vi "Wago Room PID Settings.vi"(8 "Error In":errorcluster, 10 "Wago Data Input":T2 {"Input Process Image"."Software Constants"."Room PID Settings"."Room Dehumid Temperature I (*RM Dehum I1)" max=30000 step=1; "Input Process Image"."Software Constants"."Room PID Settings"."Room Dehumid Temperature P (*RM Dehum P1)" max=30000 step=1; "Input Process Image"."Software Constants"."Room PID Settings"."Room Cool Temperature I (*RM Cool I1)" max=30000 step=1; "Input Process Image"."Software Constants"."Room PID Settings"."Room Cool Temperature P (*RM Cool P1)" max=30000 step=1; "Input Process Image"."Software Constants"."Room PID Settings"."Room Heat I (*RM Heat I1)" max=30000 step=1; "Input Process Image"."Software Constants"."Room PID Settings"."Room Heat P (*RM Heat P1)" max=30000 step=1; "Input Process Image"."Software Constants"."Room PID Settings"."Room Humidity I (*RM Hum I1)" max=30000 step=1; "Input Process Image"."Software Constants"."Room PID Settings"."Room Humidity P (*RM Hum P1)" max=30000 step=1; "Input Process Image"."Software Constants"."Room PID Settings"."Room Dry I (*RM Dry I1)" max=30000 step=1; "Input Process Image"."Software Constants"."Room PID Settings"."Room Dry P(*RM Dry P1)" max=30000 step=1}, 11 "Modbus Master in":refnum<class "Modbus Master.lvclass">) -> (0 "Error Out":errorcluster, 2 "Wago Data Output":T2 {"Input Process Image"."Software Constants"."Room PID Settings"."Room Dehumid Temperature I (*RM Dehum I1)" max=30000 step=1; "Input Process Image"."Software Constants"."Room PID Settings"."Room Dehumid Temperature P (*RM Dehum P1)" max=30000 step=1; "Input Process Image"."Software Constants"."Room PID Settings"."Room Cool Temperature I (*RM Cool I1)" max=30000 step=1; "Input Process Image"."Software Constants"."Room PID Settings"."Room Cool Temperature P (*RM Cool P1)" max=30000 step=1; "Input Process Image"."Software Constants"."Room PID Settings"."Room Heat I (*RM Heat I1)" max=30000 step=1; "Input Process Image"."Software Constants"."Room PID Settings"."Room Heat P (*RM Heat P1)" max=30000 step=1; "Input Process Image"."Software Constants"."Room PID Settings"."Room Humidity I (*RM Hum I1)" max=30000 step=1; "Input Process Image"."Software Constants"."Room PID Settings"."Room Humidity P (*RM Hum P1)" max=30000 step=1; "Input Process Image"."Software Constants"."Room PID Settings"."Room Dry I (*RM Dry I1)" max=30000 step=1; "Input Process Image"."Software Constants"."Room PID Settings"."Room Dry P(*RM Dry P1)" max=30000 step=1}, 3 "Modbus Master out":refnum<class "Modbus Master.lvclass">)   [LabVIEW 2016]
uses:
  <vilib>/NI/Modbus Library/API/Master/Modbus Master.lvclass
  Type Definitions/Wago Main Control.ctl
  Type Definitions/Wago Output Data Process Image.ctl
  Type Definitions/Wago Room Condtions.ctl
  Type Definitions/Wago Door Relays.ctl
  Type Definitions/Wago Contactor Settings.ctl
  Type Definitions/Wago Ground Leakage.ctl
  Type Definitions/Wago Input Process Image.ctl
  Type Definitions/Wago Room PID Settings.ctl
  Type Definitions/Wago Measured Input Data.ctl
  Type Definitions/Wago Room Setpoint Targets.ctl
  Type Definitions/Wago Input Commands.ctl
panel:
  in  "Ring 10":T1=344 items=["fwS1Volt1"=0, "fwS1Volt2"=1, "fwS2Volt1"=2, "fwS2Volt2"=3, "fwS3Volt1"=4, "fwS3Volt2"=5, "fwS4Volt1"=6, "fwS4Volt2"=7, "fwS5Volt1"=8, "fwS5Volt2"=9, "fwS6Volt1"=10, "fwS6Volt2 "=11, "fwS7Volt1"=12, "fwS7Volt2"=13, "fwS8Volt1"=14, "fwS8Volt2"=15, "fwRoomHum"=16, "fwRoomTemp"=17, "fwAISpare1"=18, "fwAISpare2"=19, "fwSuppTemp"=20, "fwCoolTemp"=21, "fwDehumTemp"=22, "fwUnused"=23, "Bool Inputs"=24, "gwVoltRate1"=256, "gwVoltRate2"=257, "gwVoltRate3"=258, "gwVoltRate4"=259, "gwVoltRate5"=260, "gwVoltRate6"=261, "gwVoltRate7"=262, "gwVoltRate8"=263, "gwVoltWindow5/1"=264, "gwVoltWindow6/2"=265, "gwVoltWindow7/3"=266, "gwVoltWindow8/4"=267, "fwVoltSet1"=272, "fwVoltSet2"=273, "fwVoltSet3"=274, "fwVoltSet4"=275, "fwVoltSet5"=276, "fwVoltSet6"=277, "fwVoltSet7"=278, "fwVoltSet8"=279, "fwVoltRng1"=280, "fwVoltRng2"=281, "fwVoltRng3"=282, "fwVoltRng4"=283, "fwVoltRng5"=284, "fwVoltRng6"=285, "fwVoltRng7"=286, "fwVoltRng8"=287, "fwVoltPol1"=296, "fwVoltPol2"=297, "fwVoltPol3"=298, "fwVoltPol4"=299, "fwVoltPol5"=300, "fwVoltPol6"=301, "fwVoltPol7"=302, "fwVoltPol8"=303, "Rm1St1Dr1Cmd"=304, "Rm1St2Dr1Cmd"=305, "Rm1St3Dr1Cmd"=306, "Rm1St4Dr1Cmd"=307, "Rm1St5Dr1Cmd"=308, "Rm1St6Dr1Cmd"=309, "Rm1St7Dr1Cmd"=310, "Rm1St8Dr1Cmd"=311, "Rm1St1Dr2Cmd"=312, "Rm1St2Dr2Cmd"=313, "Rm1St3Dr2Cmd"=314, "Rm1St4Dr2Cmd"=315, "Rm1St5Dr2Cmd"=316, "Rm1St6Dr2Cmd"=317, "Rm1St7Dr2Cmd"=318, "Rm1St8Dr2Cmd"=319, "Rm1St1Dr3Cmd"=320, "Rm1St2Dr3Cmd"=321, "Rm1St3Dr3Cmd"=322, "Rm1St4Dr3Cmd"=323, "Rm1St5Dr3Cmd"=324, "Rm1St6Dr3Cmd"=325, "Rm1St7Dr3Cmd"=326, "Rm1St8Dr3Cmd"=327, "fwRmTempSP"=328, "fwRmHumSP"=329, "fwCoolTempSP"=330, "fwDehumTempSP"=331, "fwRmRun"=332, "fwRmOk"=333, "fwTesting"=334, "fwRmDryP"=335, "fwRmDryI"=336, "fwRmHumP"=337, "fwRmHumI"=338, "fwRmHeatP"=339, "fwRmHeatI"=340, "fwCoolTempP"=341, "fwCoolTempI"=342, "fwDehumTempP"=343, "fwDehumTempI"=344, "fwGndLeak1"=345, "fwGndLeak2"=346, "fwGndLeak3"=347, "fwGndLeak4"=348, "fwGndLeak5"=349, "fwGndLeak6"=350, "fwGndLeak7"=351, "fwGndLeak8"=352, "Rm1OpenerCmd"=353]
  in  "Ring 9":T1=343 items=["fwS1Volt1"=0, "fwS1Volt2"=1, "fwS2Volt1"=2, "fwS2Volt2"=3, "fwS3Volt1"=4, "fwS3Volt2"=5, "fwS4Volt1"=6, "fwS4Volt2"=7, "fwS5Volt1"=8, "fwS5Volt2"=9, "fwS6Volt1"=10, "fwS6Volt2 "=11, "fwS7Volt1"=12, "fwS7Volt2"=13, "fwS8Volt1"=14, "fwS8Volt2"=15, "fwRoomHum"=16, "fwRoomTemp"=17, "fwAISpare1"=18, "fwAISpare2"=19, "fwSuppTemp"=20, "fwCoolTemp"=21, "fwDehumTemp"=22, "fwUnused"=23, "Bool Inputs"=24, "gwVoltRate1"=256, "gwVoltRate2"=257, "gwVoltRate3"=258, "gwVoltRate4"=259, "gwVoltRate5"=260, "gwVoltRate6"=261, "gwVoltRate7"=262, "gwVoltRate8"=263, "gwVoltWindow5/1"=264, "gwVoltWindow6/2"=265, "gwVoltWindow7/3"=266, "gwVoltWindow8/4"=267, "fwVoltSet1"=272, "fwVoltSet2"=273, "fwVoltSet3"=274, "fwVoltSet4"=275, "fwVoltSet5"=276, "fwVoltSet6"=277, "fwVoltSet7"=278, "fwVoltSet8"=279, "fwVoltRng1"=280, "fwVoltRng2"=281, "fwVoltRng3"=282, "fwVoltRng4"=283, "fwVoltRng5"=284, "fwVoltRng6"=285, "fwVoltRng7"=286, "fwVoltRng8"=287, "fwVoltPol1"=296, "fwVoltPol2"=297, "fwVoltPol3"=298, "fwVoltPol4"=299, "fwVoltPol5"=300, "fwVoltPol6"=301, "fwVoltPol7"=302, "fwVoltPol8"=303, "Rm1St1Dr1Cmd"=304, "Rm1St2Dr1Cmd"=305, "Rm1St3Dr1Cmd"=306, "Rm1St4Dr1Cmd"=307, "Rm1St5Dr1Cmd"=308, "Rm1St6Dr1Cmd"=309, "Rm1St7Dr1Cmd"=310, "Rm1St8Dr1Cmd"=311, "Rm1St1Dr2Cmd"=312, "Rm1St2Dr2Cmd"=313, "Rm1St3Dr2Cmd"=314, "Rm1St4Dr2Cmd"=315, "Rm1St5Dr2Cmd"=316, "Rm1St6Dr2Cmd"=317, "Rm1St7Dr2Cmd"=318, "Rm1St8Dr2Cmd"=319, "Rm1St1Dr3Cmd"=320, "Rm1St2Dr3Cmd"=321, "Rm1St3Dr3Cmd"=322, "Rm1St4Dr3Cmd"=323, "Rm1St5Dr3Cmd"=324, "Rm1St6Dr3Cmd"=325, "Rm1St7Dr3Cmd"=326, "Rm1St8Dr3Cmd"=327, "fwRmTempSP"=328, "fwRmHumSP"=329, "fwCoolTempSP"=330, "fwDehumTempSP"=331, "fwRmRun"=332, "fwRmOk"=333, "fwTesting"=334, "fwRmDryP"=335, "fwRmDryI"=336, "fwRmHumP"=337, "fwRmHumI"=338, "fwRmHeatP"=339, "fwRmHeatI"=340, "fwCoolTempP"=341, "fwCoolTempI"=342, "fwDehumTempP"=343, "fwDehumTempI"=344, "fwGndLeak1"=345, "fwGndLeak2"=346, "fwGndLeak3"=347, "fwGndLeak4"=348, "fwGndLeak5"=349, "fwGndLeak6"=350, "fwGndLeak7"=351, "fwGndLeak8"=352, "Rm1OpenerCmd"=353]
  in  "Ring 8":T1=342 items=["fwS1Volt1"=0, "fwS1Volt2"=1, "fwS2Volt1"=2, "fwS2Volt2"=3, "fwS3Volt1"=4, "fwS3Volt2"=5, "fwS4Volt1"=6, "fwS4Volt2"=7, "fwS5Volt1"=8, "fwS5Volt2"=9, "fwS6Volt1"=10, "fwS6Volt2 "=11, "fwS7Volt1"=12, "fwS7Volt2"=13, "fwS8Volt1"=14, "fwS8Volt2"=15, "fwRoomHum"=16, "fwRoomTemp"=17, "fwAISpare1"=18, "fwAISpare2"=19, "fwSuppTemp"=20, "fwCoolTemp"=21, "fwDehumTemp"=22, "fwUnused"=23, "Bool Inputs"=24, "gwVoltRate1"=256, "gwVoltRate2"=257, "gwVoltRate3"=258, "gwVoltRate4"=259, "gwVoltRate5"=260, "gwVoltRate6"=261, "gwVoltRate7"=262, "gwVoltRate8"=263, "gwVoltWindow5/1"=264, "gwVoltWindow6/2"=265, "gwVoltWindow7/3"=266, "gwVoltWindow8/4"=267, "fwVoltSet1"=272, "fwVoltSet2"=273, "fwVoltSet3"=274, "fwVoltSet4"=275, "fwVoltSet5"=276, "fwVoltSet6"=277, "fwVoltSet7"=278, "fwVoltSet8"=279, "fwVoltRng1"=280, "fwVoltRng2"=281, "fwVoltRng3"=282, "fwVoltRng4"=283, "fwVoltRng5"=284, "fwVoltRng6"=285, "fwVoltRng7"=286, "fwVoltRng8"=287, "fwVoltPol1"=296, "fwVoltPol2"=297, "fwVoltPol3"=298, "fwVoltPol4"=299, "fwVoltPol5"=300, "fwVoltPol6"=301, "fwVoltPol7"=302, "fwVoltPol8"=303, "Rm1St1Dr1Cmd"=304, "Rm1St2Dr1Cmd"=305, "Rm1St3Dr1Cmd"=306, "Rm1St4Dr1Cmd"=307, "Rm1St5Dr1Cmd"=308, "Rm1St6Dr1Cmd"=309, "Rm1St7Dr1Cmd"=310, "Rm1St8Dr1Cmd"=311, "Rm1St1Dr2Cmd"=312, "Rm1St2Dr2Cmd"=313, "Rm1St3Dr2Cmd"=314, "Rm1St4Dr2Cmd"=315, "Rm1St5Dr2Cmd"=316, "Rm1St6Dr2Cmd"=317, "Rm1St7Dr2Cmd"=318, "Rm1St8Dr2Cmd"=319, "Rm1St1Dr3Cmd"=320, "Rm1St2Dr3Cmd"=321, "Rm1St3Dr3Cmd"=322, "Rm1St4Dr3Cmd"=323, "Rm1St5Dr3Cmd"=324, "Rm1St6Dr3Cmd"=325, "Rm1St7Dr3Cmd"=326, "Rm1St8Dr3Cmd"=327, "fwRmTempSP"=328, "fwRmHumSP"=329, "fwCoolTempSP"=330, "fwDehumTempSP"=331, "fwRmRun"=332, "fwRmOk"=333, "fwTesting"=334, "fwRmDryP"=335, "fwRmDryI"=336, "fwRmHumP"=337, "fwRmHumI"=338, "fwRmHeatP"=339, "fwRmHeatI"=340, "fwCoolTempP"=341, "fwCoolTempI"=342, "fwDehumTempP"=343, "fwDehumTempI"=344, "fwGndLeak1"=345, "fwGndLeak2"=346, "fwGndLeak3"=347, "fwGndLeak4"=348, "fwGndLeak5"=349, "fwGndLeak6"=350, "fwGndLeak7"=351, "fwGndLeak8"=352, "Rm1OpenerCmd"=353]
  in  "Ring 7":T1=341 items=["fwS1Volt1"=0, "fwS1Volt2"=1, "fwS2Volt1"=2, "fwS2Volt2"=3, "fwS3Volt1"=4, "fwS3Volt2"=5, "fwS4Volt1"=6, "fwS4Volt2"=7, "fwS5Volt1"=8, "fwS5Volt2"=9, "fwS6Volt1"=10, "fwS6Volt2 "=11, "fwS7Volt1"=12, "fwS7Volt2"=13, "fwS8Volt1"=14, "fwS8Volt2"=15, "fwRoomHum"=16, "fwRoomTemp"=17, "fwAISpare1"=18, "fwAISpare2"=19, "fwSuppTemp"=20, "fwCoolTemp"=21, "fwDehumTemp"=22, "fwUnused"=23, "Bool Inputs"=24, "gwVoltRate1"=256, "gwVoltRate2"=257, "gwVoltRate3"=258, "gwVoltRate4"=259, "gwVoltRate5"=260, "gwVoltRate6"=261, "gwVoltRate7"=262, "gwVoltRate8"=263, "gwVoltWindow5/1"=264, "gwVoltWindow6/2"=265, "gwVoltWindow7/3"=266, "gwVoltWindow8/4"=267, "fwVoltSet1"=272, "fwVoltSet2"=273, "fwVoltSet3"=274, "fwVoltSet4"=275, "fwVoltSet5"=276, "fwVoltSet6"=277, "fwVoltSet7"=278, "fwVoltSet8"=279, "fwVoltRng1"=280, "fwVoltRng2"=281, "fwVoltRng3"=282, "fwVoltRng4"=283, "fwVoltRng5"=284, "fwVoltRng6"=285, "fwVoltRng7"=286, "fwVoltRng8"=287, "fwVoltPol1"=296, "fwVoltPol2"=297, "fwVoltPol3"=298, "fwVoltPol4"=299, "fwVoltPol5"=300, "fwVoltPol6"=301, "fwVoltPol7"=302, "fwVoltPol8"=303, "Rm1St1Dr1Cmd"=304, "Rm1St2Dr1Cmd"=305, "Rm1St3Dr1Cmd"=306, "Rm1St4Dr1Cmd"=307, "Rm1St5Dr1Cmd"=308, "Rm1St6Dr1Cmd"=309, "Rm1St7Dr1Cmd"=310, "Rm1St8Dr1Cmd"=311, "Rm1St1Dr2Cmd"=312, "Rm1St2Dr2Cmd"=313, "Rm1St3Dr2Cmd"=314, "Rm1St4Dr2Cmd"=315, "Rm1St5Dr2Cmd"=316, "Rm1St6Dr2Cmd"=317, "Rm1St7Dr2Cmd"=318, "Rm1St8Dr2Cmd"=319, "Rm1St1Dr3Cmd"=320, "Rm1St2Dr3Cmd"=321, "Rm1St3Dr3Cmd"=322, "Rm1St4Dr3Cmd"=323, "Rm1St5Dr3Cmd"=324, "Rm1St6Dr3Cmd"=325, "Rm1St7Dr3Cmd"=326, "Rm1St8Dr3Cmd"=327, "fwRmTempSP"=328, "fwRmHumSP"=329, "fwCoolTempSP"=330, "fwDehumTempSP"=331, "fwRmRun"=332, "fwRmOk"=333, "fwTesting"=334, "fwRmDryP"=335, "fwRmDryI"=336, "fwRmHumP"=337, "fwRmHumI"=338, "fwRmHeatP"=339, "fwRmHeatI"=340, "fwCoolTempP"=341, "fwCoolTempI"=342, "fwDehumTempP"=343, "fwDehumTempI"=344, "fwGndLeak1"=345, "fwGndLeak2"=346, "fwGndLeak3"=347, "fwGndLeak4"=348, "fwGndLeak5"=349, "fwGndLeak6"=350, "fwGndLeak7"=351, "fwGndLeak8"=352, "Rm1OpenerCmd"=353]
  in  "Ring 6":T1=340 items=["fwS1Volt1"=0, "fwS1Volt2"=1, "fwS2Volt1"=2, "fwS2Volt2"=3, "fwS3Volt1"=4, "fwS3Volt2"=5, "fwS4Volt1"=6, "fwS4Volt2"=7, "fwS5Volt1"=8, "fwS5Volt2"=9, "fwS6Volt1"=10, "fwS6Volt2 "=11, "fwS7Volt1"=12, "fwS7Volt2"=13, "fwS8Volt1"=14, "fwS8Volt2"=15, "fwRoomHum"=16, "fwRoomTemp"=17, "fwAISpare1"=18, "fwAISpare2"=19, "fwSuppTemp"=20, "fwCoolTemp"=21, "fwDehumTemp"=22, "fwUnused"=23, "Bool Inputs"=24, "gwVoltRate1"=256, "gwVoltRate2"=257, "gwVoltRate3"=258, "gwVoltRate4"=259, "gwVoltRate5"=260, "gwVoltRate6"=261, "gwVoltRate7"=262, "gwVoltRate8"=263, "gwVoltWindow5/1"=264, "gwVoltWindow6/2"=265, "gwVoltWindow7/3"=266, "gwVoltWindow8/4"=267, "fwVoltSet1"=272, "fwVoltSet2"=273, "fwVoltSet3"=274, "fwVoltSet4"=275, "fwVoltSet5"=276, "fwVoltSet6"=277, "fwVoltSet7"=278, "fwVoltSet8"=279, "fwVoltRng1"=280, "fwVoltRng2"=281, "fwVoltRng3"=282, "fwVoltRng4"=283, "fwVoltRng5"=284, "fwVoltRng6"=285, "fwVoltRng7"=286, "fwVoltRng8"=287, "fwVoltPol1"=296, "fwVoltPol2"=297, "fwVoltPol3"=298, "fwVoltPol4"=299, "fwVoltPol5"=300, "fwVoltPol6"=301, "fwVoltPol7"=302, "fwVoltPol8"=303, "Rm1St1Dr1Cmd"=304, "Rm1St2Dr1Cmd"=305, "Rm1St3Dr1Cmd"=306, "Rm1St4Dr1Cmd"=307, "Rm1St5Dr1Cmd"=308, "Rm1St6Dr1Cmd"=309, "Rm1St7Dr1Cmd"=310, "Rm1St8Dr1Cmd"=311, "Rm1St1Dr2Cmd"=312, "Rm1St2Dr2Cmd"=313, "Rm1St3Dr2Cmd"=314, "Rm1St4Dr2Cmd"=315, "Rm1St5Dr2Cmd"=316, "Rm1St6Dr2Cmd"=317, "Rm1St7Dr2Cmd"=318, "Rm1St8Dr2Cmd"=319, "Rm1St1Dr3Cmd"=320, "Rm1St2Dr3Cmd"=321, "Rm1St3Dr3Cmd"=322, "Rm1St4Dr3Cmd"=323, "Rm1St5Dr3Cmd"=324, "Rm1St6Dr3Cmd"=325, "Rm1St7Dr3Cmd"=326, "Rm1St8Dr3Cmd"=327, "fwRmTempSP"=328, "fwRmHumSP"=329, "fwCoolTempSP"=330, "fwDehumTempSP"=331, "fwRmRun"=332, "fwRmOk"=333, "fwTesting"=334, "fwRmDryP"=335, "fwRmDryI"=336, "fwRmHumP"=337, "fwRmHumI"=338, "fwRmHeatP"=339, "fwRmHeatI"=340, "fwCoolTempP"=341, "fwCoolTempI"=342, "fwDehumTempP"=343, "fwDehumTempI"=344, "fwGndLeak1"=345, "fwGndLeak2"=346, "fwGndLeak3"=347, "fwGndLeak4"=348, "fwGndLeak5"=349, "fwGndLeak6"=350, "fwGndLeak7"=351, "fwGndLeak8"=352, "Rm1OpenerCmd"=353]
  in  "Ring 5":T1=339 items=["fwS1Volt1"=0, "fwS1Volt2"=1, "fwS2Volt1"=2, "fwS2Volt2"=3, "fwS3Volt1"=4, "fwS3Volt2"=5, "fwS4Volt1"=6, "fwS4Volt2"=7, "fwS5Volt1"=8, "fwS5Volt2"=9, "fwS6Volt1"=10, "fwS6Volt2 "=11, "fwS7Volt1"=12, "fwS7Volt2"=13, "fwS8Volt1"=14, "fwS8Volt2"=15, "fwRoomHum"=16, "fwRoomTemp"=17, "fwAISpare1"=18, "fwAISpare2"=19, "fwSuppTemp"=20, "fwCoolTemp"=21, "fwDehumTemp"=22, "fwUnused"=23, "Bool Inputs"=24, "gwVoltRate1"=256, "gwVoltRate2"=257, "gwVoltRate3"=258, "gwVoltRate4"=259, "gwVoltRate5"=260, "gwVoltRate6"=261, "gwVoltRate7"=262, "gwVoltRate8"=263, "gwVoltWindow5/1"=264, "gwVoltWindow6/2"=265, "gwVoltWindow7/3"=266, "gwVoltWindow8/4"=267, "fwVoltSet1"=272, "fwVoltSet2"=273, "fwVoltSet3"=274, "fwVoltSet4"=275, "fwVoltSet5"=276, "fwVoltSet6"=277, "fwVoltSet7"=278, "fwVoltSet8"=279, "fwVoltRng1"=280, "fwVoltRng2"=281, "fwVoltRng3"=282, "fwVoltRng4"=283, "fwVoltRng5"=284, "fwVoltRng6"=285, "fwVoltRng7"=286, "fwVoltRng8"=287, "fwVoltPol1"=296, "fwVoltPol2"=297, "fwVoltPol3"=298, "fwVoltPol4"=299, "fwVoltPol5"=300, "fwVoltPol6"=301, "fwVoltPol7"=302, "fwVoltPol8"=303, "Rm1St1Dr1Cmd"=304, "Rm1St2Dr1Cmd"=305, "Rm1St3Dr1Cmd"=306, "Rm1St4Dr1Cmd"=307, "Rm1St5Dr1Cmd"=308, "Rm1St6Dr1Cmd"=309, "Rm1St7Dr1Cmd"=310, "Rm1St8Dr1Cmd"=311, "Rm1St1Dr2Cmd"=312, "Rm1St2Dr2Cmd"=313, "Rm1St3Dr2Cmd"=314, "Rm1St4Dr2Cmd"=315, "Rm1St5Dr2Cmd"=316, "Rm1St6Dr2Cmd"=317, "Rm1St7Dr2Cmd"=318, "Rm1St8Dr2Cmd"=319, "Rm1St1Dr3Cmd"=320, "Rm1St2Dr3Cmd"=321, "Rm1St3Dr3Cmd"=322, "Rm1St4Dr3Cmd"=323, "Rm1St5Dr3Cmd"=324, "Rm1St6Dr3Cmd"=325, "Rm1St7Dr3Cmd"=326, "Rm1St8Dr3Cmd"=327, "fwRmTempSP"=328, "fwRmHumSP"=329, "fwCoolTempSP"=330, "fwDehumTempSP"=331, "fwRmRun"=332, "fwRmOk"=333, "fwTesting"=334, "fwRmDryP"=335, "fwRmDryI"=336, "fwRmHumP"=337, "fwRmHumI"=338, "fwRmHeatP"=339, "fwRmHeatI"=340, "fwCoolTempP"=341, "fwCoolTempI"=342, "fwDehumTempP"=343, "fwDehumTempI"=344, "fwGndLeak1"=345, "fwGndLeak2"=346, "fwGndLeak3"=347, "fwGndLeak4"=348, "fwGndLeak5"=349, "fwGndLeak6"=350, "fwGndLeak7"=351, "fwGndLeak8"=352, "Rm1OpenerCmd"=353]
  in  "Ring 4":T1=338 items=["fwS1Volt1"=0, "fwS1Volt2"=1, "fwS2Volt1"=2, "fwS2Volt2"=3, "fwS3Volt1"=4, "fwS3Volt2"=5, "fwS4Volt1"=6, "fwS4Volt2"=7, "fwS5Volt1"=8, "fwS5Volt2"=9, "fwS6Volt1"=10, "fwS6Volt2 "=11, "fwS7Volt1"=12, "fwS7Volt2"=13, "fwS8Volt1"=14, "fwS8Volt2"=15, "fwRoomHum"=16, "fwRoomTemp"=17, "fwAISpare1"=18, "fwAISpare2"=19, "fwSuppTemp"=20, "fwCoolTemp"=21, "fwDehumTemp"=22, "fwUnused"=23, "Bool Inputs"=24, "gwVoltRate1"=256, "gwVoltRate2"=257, "gwVoltRate3"=258, "gwVoltRate4"=259, "gwVoltRate5"=260, "gwVoltRate6"=261, "gwVoltRate7"=262, "gwVoltRate8"=263, "gwVoltWindow5/1"=264, "gwVoltWindow6/2"=265, "gwVoltWindow7/3"=266, "gwVoltWindow8/4"=267, "fwVoltSet1"=272, "fwVoltSet2"=273, "fwVoltSet3"=274, "fwVoltSet4"=275, "fwVoltSet5"=276, "fwVoltSet6"=277, "fwVoltSet7"=278, "fwVoltSet8"=279, "fwVoltRng1"=280, "fwVoltRng2"=281, "fwVoltRng3"=282, "fwVoltRng4"=283, "fwVoltRng5"=284, "fwVoltRng6"=285, "fwVoltRng7"=286, "fwVoltRng8"=287, "fwVoltPol1"=296, "fwVoltPol2"=297, "fwVoltPol3"=298, "fwVoltPol4"=299, "fwVoltPol5"=300, "fwVoltPol6"=301, "fwVoltPol7"=302, "fwVoltPol8"=303, "Rm1St1Dr1Cmd"=304, "Rm1St2Dr1Cmd"=305, "Rm1St3Dr1Cmd"=306, "Rm1St4Dr1Cmd"=307, "Rm1St5Dr1Cmd"=308, "Rm1St6Dr1Cmd"=309, "Rm1St7Dr1Cmd"=310, "Rm1St8Dr1Cmd"=311, "Rm1St1Dr2Cmd"=312, "Rm1St2Dr2Cmd"=313, "Rm1St3Dr2Cmd"=314, "Rm1St4Dr2Cmd"=315, "Rm1St5Dr2Cmd"=316, "Rm1St6Dr2Cmd"=317, "Rm1St7Dr2Cmd"=318, "Rm1St8Dr2Cmd"=319, "Rm1St1Dr3Cmd"=320, "Rm1St2Dr3Cmd"=321, "Rm1St3Dr3Cmd"=322, "Rm1St4Dr3Cmd"=323, "Rm1St5Dr3Cmd"=324, "Rm1St6Dr3Cmd"=325, "Rm1St7Dr3Cmd"=326, "Rm1St8Dr3Cmd"=327, "fwRmTempSP"=328, "fwRmHumSP"=329, "fwCoolTempSP"=330, "fwDehumTempSP"=331, "fwRmRun"=332, "fwRmOk"=333, "fwTesting"=334, "fwRmDryP"=335, "fwRmDryI"=336, "fwRmHumP"=337, "fwRmHumI"=338, "fwRmHeatP"=339, "fwRmHeatI"=340, "fwCoolTempP"=341, "fwCoolTempI"=342, "fwDehumTempP"=343, "fwDehumTempI"=344, "fwGndLeak1"=345, "fwGndLeak2"=346, "fwGndLeak3"=347, "fwGndLeak4"=348, "fwGndLeak5"=349, "fwGndLeak6"=350, "fwGndLeak7"=351, "fwGndLeak8"=352, "Rm1OpenerCmd"=353]
  in  "Ring 3":T1=337 items=["fwS1Volt1"=0, "fwS1Volt2"=1, "fwS2Volt1"=2, "fwS2Volt2"=3, "fwS3Volt1"=4, "fwS3Volt2"=5, "fwS4Volt1"=6, "fwS4Volt2"=7, "fwS5Volt1"=8, "fwS5Volt2"=9, "fwS6Volt1"=10, "fwS6Volt2 "=11, "fwS7Volt1"=12, "fwS7Volt2"=13, "fwS8Volt1"=14, "fwS8Volt2"=15, "fwRoomHum"=16, "fwRoomTemp"=17, "fwAISpare1"=18, "fwAISpare2"=19, "fwSuppTemp"=20, "fwCoolTemp"=21, "fwDehumTemp"=22, "fwUnused"=23, "Bool Inputs"=24, "gwVoltRate1"=256, "gwVoltRate2"=257, "gwVoltRate3"=258, "gwVoltRate4"=259, "gwVoltRate5"=260, "gwVoltRate6"=261, "gwVoltRate7"=262, "gwVoltRate8"=263, "gwVoltWindow5/1"=264, "gwVoltWindow6/2"=265, "gwVoltWindow7/3"=266, "gwVoltWindow8/4"=267, "fwVoltSet1"=272, "fwVoltSet2"=273, "fwVoltSet3"=274, "fwVoltSet4"=275, "fwVoltSet5"=276, "fwVoltSet6"=277, "fwVoltSet7"=278, "fwVoltSet8"=279, "fwVoltRng1"=280, "fwVoltRng2"=281, "fwVoltRng3"=282, "fwVoltRng4"=283, "fwVoltRng5"=284, "fwVoltRng6"=285, "fwVoltRng7"=286, "fwVoltRng8"=287, "fwVoltPol1"=296, "fwVoltPol2"=297, "fwVoltPol3"=298, "fwVoltPol4"=299, "fwVoltPol5"=300, "fwVoltPol6"=301, "fwVoltPol7"=302, "fwVoltPol8"=303, "Rm1St1Dr1Cmd"=304, "Rm1St2Dr1Cmd"=305, "Rm1St3Dr1Cmd"=306, "Rm1St4Dr1Cmd"=307, "Rm1St5Dr1Cmd"=308, "Rm1St6Dr1Cmd"=309, "Rm1St7Dr1Cmd"=310, "Rm1St8Dr1Cmd"=311, "Rm1St1Dr2Cmd"=312, "Rm1St2Dr2Cmd"=313, "Rm1St3Dr2Cmd"=314, "Rm1St4Dr2Cmd"=315, "Rm1St5Dr2Cmd"=316, "Rm1St6Dr2Cmd"=317, "Rm1St7Dr2Cmd"=318, "Rm1St8Dr2Cmd"=319, "Rm1St1Dr3Cmd"=320, "Rm1St2Dr3Cmd"=321, "Rm1St3Dr3Cmd"=322, "Rm1St4Dr3Cmd"=323, "Rm1St5Dr3Cmd"=324, "Rm1St6Dr3Cmd"=325, "Rm1St7Dr3Cmd"=326, "Rm1St8Dr3Cmd"=327, "fwRmTempSP"=328, "fwRmHumSP"=329, "fwCoolTempSP"=330, "fwDehumTempSP"=331, "fwRmRun"=332, "fwRmOk"=333, "fwTesting"=334, "fwRmDryP"=335, "fwRmDryI"=336, "fwRmHumP"=337, "fwRmHumI"=338, "fwRmHeatP"=339, "fwRmHeatI"=340, "fwCoolTempP"=341, "fwCoolTempI"=342, "fwDehumTempP"=343, "fwDehumTempI"=344, "fwGndLeak1"=345, "fwGndLeak2"=346, "fwGndLeak3"=347, "fwGndLeak4"=348, "fwGndLeak5"=349, "fwGndLeak6"=350, "fwGndLeak7"=351, "fwGndLeak8"=352, "Rm1OpenerCmd"=353]
  in  "Ring 2":T1=336 items=["fwS1Volt1"=0, "fwS1Volt2"=1, "fwS2Volt1"=2, "fwS2Volt2"=3, "fwS3Volt1"=4, "fwS3Volt2"=5, "fwS4Volt1"=6, "fwS4Volt2"=7, "fwS5Volt1"=8, "fwS5Volt2"=9, "fwS6Volt1"=10, "fwS6Volt2 "=11, "fwS7Volt1"=12, "fwS7Volt2"=13, "fwS8Volt1"=14, "fwS8Volt2"=15, "fwRoomHum"=16, "fwRoomTemp"=17, "fwAISpare1"=18, "fwAISpare2"=19, "fwSuppTemp"=20, "fwCoolTemp"=21, "fwDehumTemp"=22, "fwUnused"=23, "Bool Inputs"=24, "gwVoltRate1"=256, "gwVoltRate2"=257, "gwVoltRate3"=258, "gwVoltRate4"=259, "gwVoltRate5"=260, "gwVoltRate6"=261, "gwVoltRate7"=262, "gwVoltRate8"=263, "gwVoltWindow5/1"=264, "gwVoltWindow6/2"=265, "gwVoltWindow7/3"=266, "gwVoltWindow8/4"=267, "fwVoltSet1"=272, "fwVoltSet2"=273, "fwVoltSet3"=274, "fwVoltSet4"=275, "fwVoltSet5"=276, "fwVoltSet6"=277, "fwVoltSet7"=278, "fwVoltSet8"=279, "fwVoltRng1"=280, "fwVoltRng2"=281, "fwVoltRng3"=282, "fwVoltRng4"=283, "fwVoltRng5"=284, "fwVoltRng6"=285, "fwVoltRng7"=286, "fwVoltRng8"=287, "fwVoltPol1"=296, "fwVoltPol2"=297, "fwVoltPol3"=298, "fwVoltPol4"=299, "fwVoltPol5"=300, "fwVoltPol6"=301, "fwVoltPol7"=302, "fwVoltPol8"=303, "Rm1St1Dr1Cmd"=304, "Rm1St2Dr1Cmd"=305, "Rm1St3Dr1Cmd"=306, "Rm1St4Dr1Cmd"=307, "Rm1St5Dr1Cmd"=308, "Rm1St6Dr1Cmd"=309, "Rm1St7Dr1Cmd"=310, "Rm1St8Dr1Cmd"=311, "Rm1St1Dr2Cmd"=312, "Rm1St2Dr2Cmd"=313, "Rm1St3Dr2Cmd"=314, "Rm1St4Dr2Cmd"=315, "Rm1St5Dr2Cmd"=316, "Rm1St6Dr2Cmd"=317, "Rm1St7Dr2Cmd"=318, "Rm1St8Dr2Cmd"=319, "Rm1St1Dr3Cmd"=320, "Rm1St2Dr3Cmd"=321, "Rm1St3Dr3Cmd"=322, "Rm1St4Dr3Cmd"=323, "Rm1St5Dr3Cmd"=324, "Rm1St6Dr3Cmd"=325, "Rm1St7Dr3Cmd"=326, "Rm1St8Dr3Cmd"=327, "fwRmTempSP"=328, "fwRmHumSP"=329, "fwCoolTempSP"=330, "fwDehumTempSP"=331, "fwRmRun"=332, "fwRmOk"=333, "fwTesting"=334, "fwRmDryP"=335, "fwRmDryI"=336, "fwRmHumP"=337, "fwRmHumI"=338, "fwRmHeatP"=339, "fwRmHeatI"=340, "fwCoolTempP"=341, "fwCoolTempI"=342, "fwDehumTempP"=343, "fwDehumTempI"=344, "fwGndLeak1"=345, "fwGndLeak2"=346, "fwGndLeak3"=347, "fwGndLeak4"=348, "fwGndLeak5"=349, "fwGndLeak6"=350, "fwGndLeak7"=351, "fwGndLeak8"=352, "Rm1OpenerCmd"=353]
  in  "Ring":T1=335 items=["fwS1Volt1"=0, "fwS1Volt2"=1, "fwS2Volt1"=2, "fwS2Volt2"=3, "fwS3Volt1"=4, "fwS3Volt2"=5, "fwS4Volt1"=6, "fwS4Volt2"=7, "fwS5Volt1"=8, "fwS5Volt2"=9, "fwS6Volt1"=10, "fwS6Volt2 "=11, "fwS7Volt1"=12, "fwS7Volt2"=13, "fwS8Volt1"=14, "fwS8Volt2"=15, "fwRoomHum"=16, "fwRoomTemp"=17, "fwAISpare1"=18, "fwAISpare2"=19, "fwSuppTemp"=20, "fwCoolTemp"=21, "fwDehumTemp"=22, "fwUnused"=23, "Bool Inputs"=24, "gwVoltRate1"=256, "gwVoltRate2"=257, "gwVoltRate3"=258, "gwVoltRate4"=259, "gwVoltRate5"=260, "gwVoltRate6"=261, "gwVoltRate7"=262, "gwVoltRate8"=263, "gwVoltWindow5/1"=264, "gwVoltWindow6/2"=265, "gwVoltWindow7/3"=266, "gwVoltWindow8/4"=267, "fwVoltSet1"=272, "fwVoltSet2"=273, "fwVoltSet3"=274, "fwVoltSet4"=275, "fwVoltSet5"=276, "fwVoltSet6"=277, "fwVoltSet7"=278, "fwVoltSet8"=279, "fwVoltRng1"=280, "fwVoltRng2"=281, "fwVoltRng3"=282, "fwVoltRng4"=283, "fwVoltRng5"=284, "fwVoltRng6"=285, "fwVoltRng7"=286, "fwVoltRng8"=287, "fwVoltPol1"=296, "fwVoltPol2"=297, "fwVoltPol3"=298, "fwVoltPol4"=299, "fwVoltPol5"=300, "fwVoltPol6"=301, "fwVoltPol7"=302, "fwVoltPol8"=303, "Rm1St1Dr1Cmd"=304, "Rm1St2Dr1Cmd"=305, "Rm1St3Dr1Cmd"=306, "Rm1St4Dr1Cmd"=307, "Rm1St5Dr1Cmd"=308, "Rm1St6Dr1Cmd"=309, "Rm1St7Dr1Cmd"=310, "Rm1St8Dr1Cmd"=311, "Rm1St1Dr2Cmd"=312, "Rm1St2Dr2Cmd"=313, "Rm1St3Dr2Cmd"=314, "Rm1St4Dr2Cmd"=315, "Rm1St5Dr2Cmd"=316, "Rm1St6Dr2Cmd"=317, "Rm1St7Dr2Cmd"=318, "Rm1St8Dr2Cmd"=319, "Rm1St1Dr3Cmd"=320, "Rm1St2Dr3Cmd"=321, "Rm1St3Dr3Cmd"=322, "Rm1St4Dr3Cmd"=323, "Rm1St5Dr3Cmd"=324, "Rm1St6Dr3Cmd"=325, "Rm1St7Dr3Cmd"=326, "Rm1St8Dr3Cmd"=327, "fwRmTempSP"=328, "fwRmHumSP"=329, "fwCoolTempSP"=330, "fwDehumTempSP"=331, "fwRmRun"=332, "fwRmOk"=333, "fwTesting"=334, "fwRmDryP"=335, "fwRmDryI"=336, "fwRmHumP"=337, "fwRmHumI"=338, "fwRmHeatP"=339, "fwRmHeatI"=340, "fwCoolTempP"=341, "fwCoolTempI"=342, "fwDehumTempP"=343, "fwDehumTempI"=344, "fwGndLeak1"=345, "fwGndLeak2"=346, "fwGndLeak3"=347, "fwGndLeak4"=348, "fwGndLeak5"=349, "fwGndLeak6"=350, "fwGndLeak7"=351, "fwGndLeak8"=352, "Rm1OpenerCmd"=353]
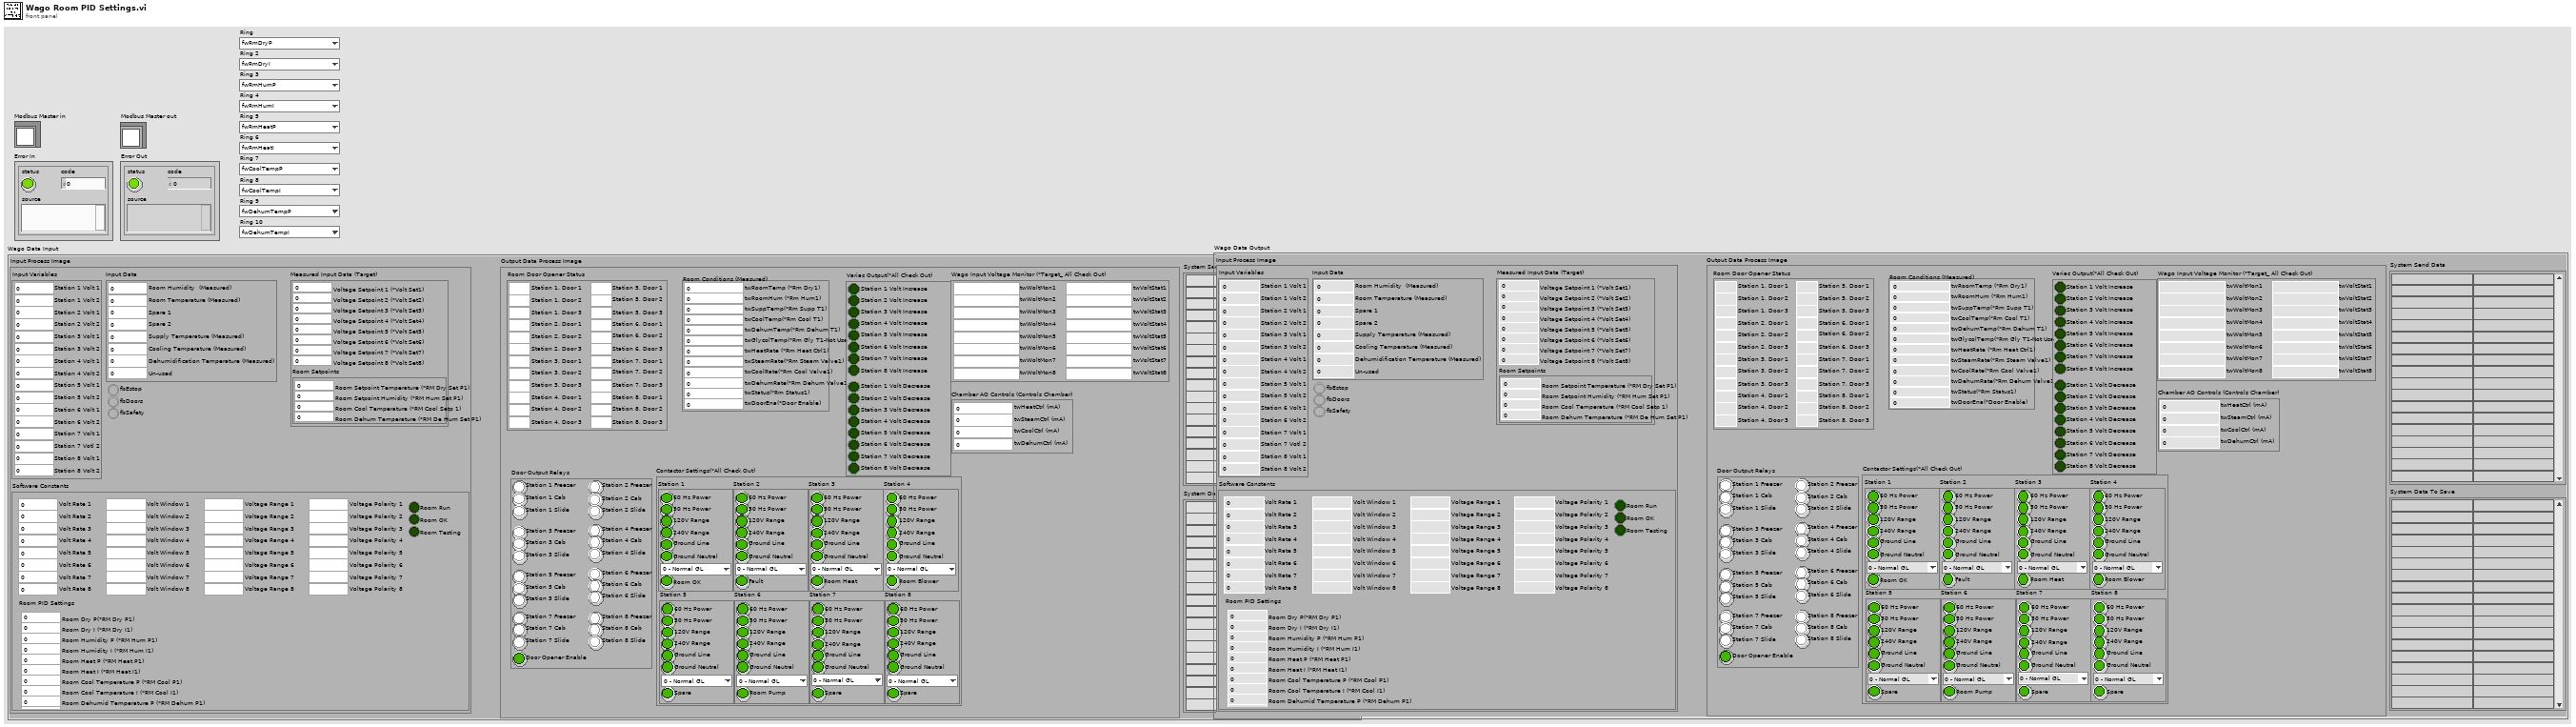
[diagram p1: front panel]
types:
  T1 = typedef "Wago Input Commands.ctl" = u16
  T2 = typedef "Wago Main Control.ctl" = cluster{"Output Data Process Image":T3, "Input Process Image":T8, "System Send Data":string[][], "System Data To Save":string[][]}
  T3 = typedef "Wago Output Data Process Image.ctl" = cluster{"Room Door Opener Status":cluster{"Station 1, Door 1":u16, "Station 1, Door 2":u16, "Station 1, Door 3":u16, "Station 2, Door 1":u16, "Station 2, Door 2":u16, "Station 2, Door 3":u16, "Station 3, Door 1":u16, "Station 3, Door 2":u16, "Station 3, Door 3":u16, "Station 4, Door 1":u16, "Station 4, Door 2":u16, "Station 4, Door 3":u16, "Station 5, Door 1":u16, "Station 5, Door 2":u16, "Station 5, Door 3":u16, "Station 6, Door 1":u16, "Station 6, Door 2":u16, "Station 6, Door 3":u16, "Station 7, Door 1":u16, "Station 7, Door 2":u16, "Station 7, Door 3":u16, "Station 8, Door 1":u16, "Station 8, Door 2":u16, "Station 8, Door 3":u16}, "Room Conditions (Measured)":T4, "Chamber AO Controls (Controls Chamber)":cluster{"twDehumCtrl (mA)":u16, "twCoolCtrl (mA)":u16, "twSteamCtrl (mA)":u16, "twHeatCtrl (mA)":u16}, "Variac Output(*All Check Out)":cluster{"Station 1 Volt Increase":bool, "Station 1 Volt Decrease":bool, "Station 2 Volt Increase":bool, "Station 2 Volt Decrease":bool, "Station 3 Volt Increase":bool, "Station 3 Volt Decrease":bool, "Station 4 Volt Increase":bool, "Station 4 Volt Decrease":bool, "Station 5 Volt Increase":bool, "Station 5 Volt Decrease":bool, "Station 6 Volt Increase":bool, "Station 6 Volt Decrease":bool, "Station 7 Volt Increase":bool, "Station 7 Volt Decrease":bool, "Station 8 Volt Increase":bool, "Station 8 Volt Decrease":bool}, "Door Output Relays":T5, "Wago Input Voltage Monitor (*Target_ All Check Out)":cluster{"twWoltMon1":dbl, "twWoltMon2":dbl, "twWoltMon3":dbl, "twWoltMon4":dbl, "twWoltMon5":dbl, "twWoltMon6":dbl, "twWoltMon7":dbl, "twWoltMon8":dbl, "twVoltStat1":u16, "twVoltStat2":u16, "twVoltStat3":u16, "twVoltStat4":u16, "twVoltStat5":u16, "twVoltStat6":u16, "twVoltStat7":u16, "twVoltStat8":u16}, "Contactor Settings(*All Check Out)":T6}
  T4 = typedef "Wago Room Condtions.ctl" = cluster{"twDoorEna(*Door Enable)":u16, "twStatus(*Rm Status1)":u16, "twRoomTemp (*Rm Dry1)":dbl, "twRoomHum (*Rm Hum1)":dbl, "twSuppTemp(*Rm Supp T1)":dbl, "twCoolTemp(*Rm Cool T1)":dbl, "twDehumTemp(*Rm Dehum T1)":dbl, "twGlycolTemp(*Rm Gly T1-Not Used)":dbl, "twDehumRate(*Rm Dehum Valve1)":dbl, "twCoolRate(*Rm Cool Valve1)":dbl, "twSteamRate(*Rm Steam Valve1)":dbl, "twHeatRate (*Rm Heat Ctrl1)":dbl}
  T5 = typedef "Wago Door Relays.ctl" = cluster{"Station 1 Freezer":bool, "Station 1 Cab":bool, "Station 1 Slide":bool, "Station 2 Freezer":bool, "Station 2 Cab":bool, "Station 2 Slide":bool, "Station 3 Freezer":bool, "Station 3 Cab":bool, "Station 3 Slide":bool, "Station 4 Freezer":bool, "Station 4 Cab":bool, "Station 4 Slide":bool, "Station 5 Freezer":bool, "Station 5 Cab":bool, "Station 5 Slide":bool, "Station 6 Freezer":bool, "Station 6 Cab":bool, "Station 6 Slide":bool, "Station 7 Freezer":bool, "Station 7 Cab":bool, "Station 7 Slide":bool, "Station 8 Freezer":bool, "Station 8 Cab":bool, "Station 8 Slide":bool, "Door Opener Enable":bool}
  T6 = typedef "Wago Contactor Settings.ctl" = cluster{"Station 1":cluster{"60 Hz Power":bool, "50 Hz Power":bool, "120V Range":bool, "240V Range":bool, "Ground Line":bool, "Ground Neutral":bool, "Room OK":bool, "Ground Leakage":T7}, "Station 2":cluster{"60 Hz Power":bool, "50 Hz Power":bool, "120V Range":bool, "240V Range":bool, "Ground Line":bool, "Ground Neutral":bool, "Fault":bool, "Ground Leakage":T7}, "Station 3":cluster{"60 Hz Power":bool, "50 Hz Power":bool, "120V Range":bool, "240V Range":bool, "Ground Line":bool, "Ground Neutral":bool, "Room Heat":bool, "Ground Leakage":T7}, "Station 4":cluster{"60 Hz Power":bool, "50 Hz Power":bool, "120V Range":bool, "240V Range":bool, "Ground Line":bool, "Ground Neutral":bool, "Room Blower":bool, "Ground Leakage":T7}, "Station 5":cluster{"60 Hz Power":bool, "50 Hz Power":bool, "120V Range":bool, "240V Range":bool, "Ground Line":bool, "Ground Neutral":bool, "Spare":bool, "Ground Leakage":T7}, "Station 6":cluster{"60 Hz Power":bool, "50 Hz Power":bool, "120V Range":bool, "240V Range":bool, "Ground Line":bool, "Ground Neutral":bool, "Room Pump":bool, "Ground Leakage":T7}, "Station 7":cluster{"60 Hz Power":bool, "50 Hz Power":bool, "120V Range":bool, "240V Range":bool, "Ground Line":bool, "Ground Neutral":bool, "Spare":bool, "Ground Leakage":T7}, "Station 8":cluster{"60 Hz Power":bool, "50 Hz Power":bool, "120V Range":bool, "240V Range":bool, "Ground Line":bool, "Ground Neutral":bool, "Spare":bool, "Ground Leakage":T7}}
  T7 = typedef "Wago Ground Leakage.ctl" = enum16{"0 - Normal GL", "1 - Measure GL"}
  T8 = typedef "Wago Input Process Image.ctl" = cluster{"fbEstop":bool, "fbDoors":bool, "fbSafety":bool, "Input Variables":cluster{"Station 1 Volt 1":dbl, "Station 1 Volt 2":dbl, "Station 2 Volt 1":dbl, "Station 2 Volt 2":dbl, "Station 3 Volt 1":dbl, "Station 3 Volt 2":dbl, "Station 4 Volt 1":dbl, "Station 4 Volt 2":dbl, "Station 5 Volt 1":dbl, "Station 5 Volt 2":dbl, "Station 6 Volt 1":dbl, "Station 6 Volt 2":dbl, "Station 7 Volt 1":dbl, "Station 7 Votl 2":dbl, "Station 8 Volt 1":dbl, "Station 8 Volt 2":dbl}, "Input Data":cluster{"Room Humidity  (Measured)":dbl, "Room Temperature (Measured)":dbl, "Spare 1":dbl, "Spare 2":dbl, "Supply Temperature (Measured)":dbl, "Cooling Temperature (Measured)":dbl, "Dehumidification Temperature (Measured)":dbl, "Un-used":dbl}, "Software Constants":cluster{"Volt Rate 1":u16, "Volt Rate 2":u16, "Volt Rate 3":u16, "Volt Rate 4":u16, "Volt Rate 5":u16, "Volt Rate 6":u16, "Volt Rate 7":u16, "Volt Rate 8":u16, "Volt Window 1":u16, "Volt Window 2":u16, "Volt Window 3":u16, "Volt Window 4":u16, "Volt Window 5":u16, "Volt Window 6":u16, "Volt Window 7":u16, "Volt Window 8":u16, "Voltage Range 1":u16, "Voltage Range 2":u16, "Voltage Range 3":u16, "Voltage Range 4":u16, "Voltage Range 5":u16, "Voltage Range 6":u16, "Voltage Range 7":u16, "Voltage Range 8":u16, "Voltage Polarity 1":u16, "Voltage Polarity 2":u16, "Voltage Polarity 3":u16, "Voltage Polarity 4":u16, "Voltage Polarity 5":u16, "Voltage Polarity 6":u16, "Voltage Polarity 7":u16, "Voltage Polarity 8":u16, "Room Run":bool, "Room OK":bool, "Room Testing":bool, "Room PID Settings":T9}, "Measured Input Data (Target)":T10}
  T9 = typedef "Wago Room PID Settings.ctl" = cluster{"Room Dry P(*RM Dry P1)":u16, "Room Dry I (*RM Dry I1)":u16, "Room Humidity P (*RM Hum P1)":u16, "Room Humidity I (*RM Hum I1)":u16, "Room Heat P (*RM Heat P1)":u16, "Room Heat I (*RM Heat I1)":u16, "Room Cool Temperature P (*RM Cool P1)":u16, "Room Cool Temperature I (*RM Cool I1)":u16, "Room Dehumid Temperature P (*RM Dehum P1)":u16, "Room Dehumid Temperature I (*RM Dehum I1)":u16}
  T10 = typedef "Wago Measured Input Data.ctl" = cluster{"Voltage Setpoint 1 (*Volt Set1)":dbl, "Voltage Setpoint 2 (*Volt Set2)":dbl, "Voltage Setpoint 3 (*Volt Set3)":dbl, "Voltage Setpoint 4 (*Volt Set4)":dbl, "Voltage Setpoint 5 (*Volt Set5)":dbl, "Voltage Setpoint 6 (*Volt Set6)":dbl, "Voltage Setpoint 7 (*Volt Set7)":dbl, "Voltage Setpoint 8 (*Volt Set8)":dbl, "Room Setpoints":T11}
  T11 = typedef "Wago Room Setpoint Targets.ctl" = cluster{"Room Setpoint Temperature (*RM Dry Set P1)":dbl, "Room Setpoint Humidity (*RM Hum Set P1)":dbl, "Room Cool Temperature (*RM Cool Setp 1)":dbl, "Room Dehum Temperature (*RM De Hum Set P1)":dbl}
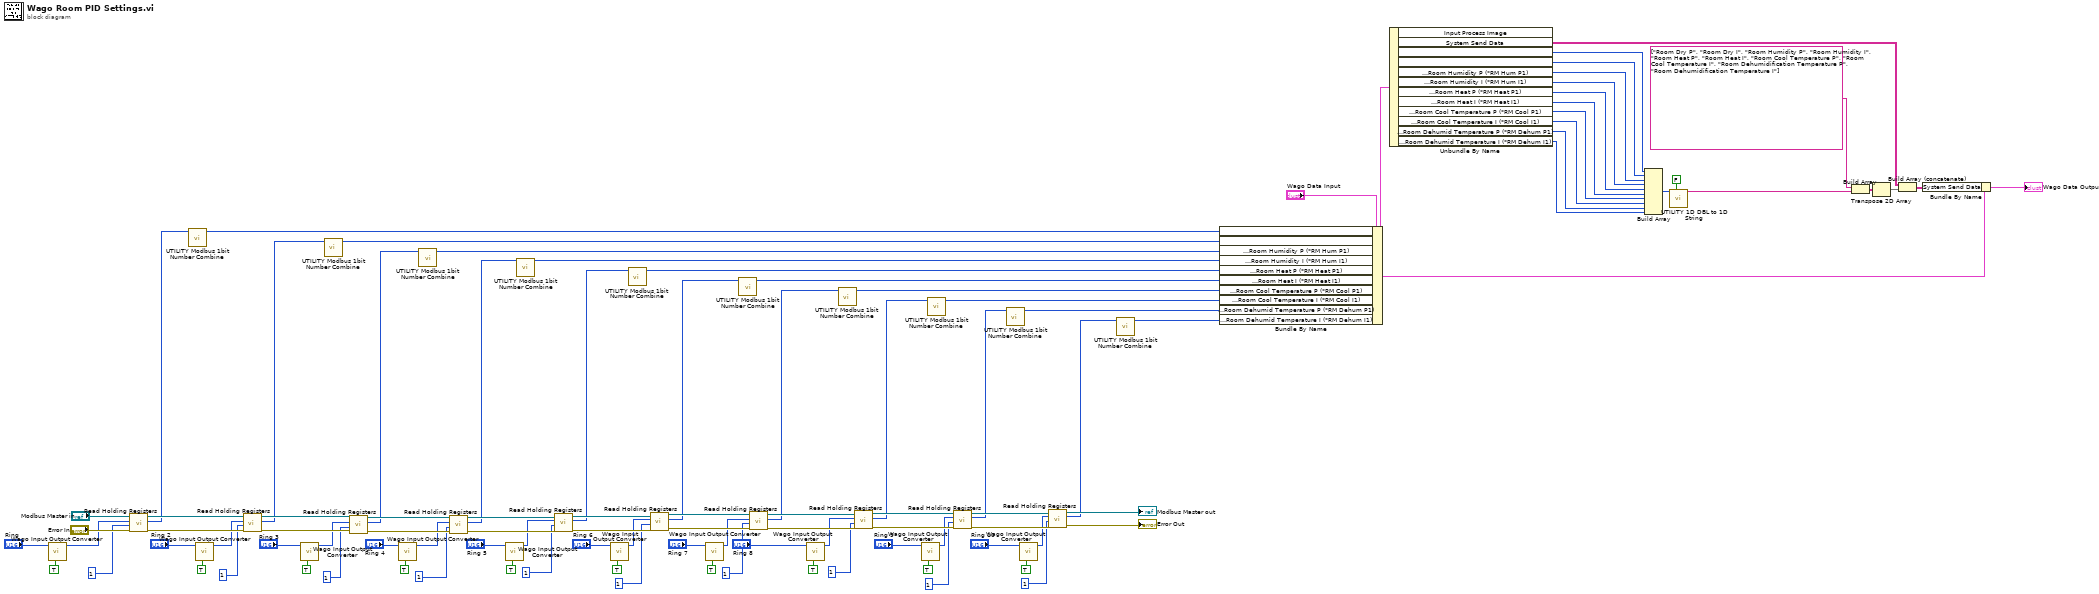
[diagram p0: block diagram]
diagram:
  n1 = call "Wago Input Output Converter.vi"("Input to Output?"=TRUE, "Input Command"="Ring") -> ("Read Input Command Location"=w68:i32)  [unwired: 9 in]
  n2 = call-dynamic "Read Holding Registers.vi"("error in"="Error In", "number of inputs"=u16 1, "starting address"=w68, "Modbus master in"="Modbus Master in") -> ("error out"=w103:errorcluster, "register values"=w40:u16[], "Modbus master out"=w87:refnum<class "Modbus Master.lvclass">)  [unwired: 5 in]
  n3 = call "UTILITY Modbus 1bit Number Combine.vi"("register values"=w40) -> ("Data"=w31:u16)  [unwired: 10 in]
  n4 = call "Wago Input Output Converter.vi"("Input to Output?"=TRUE, "Input Command"="Ring 2") -> ("Read Input Command Location"=w65:i32)  [unwired: 9 in]
  n5 = call-dynamic "Read Holding Registers.vi"("error in"=w103, "number of inputs"=u16 1, "starting address"=w65, "Modbus master in"=w87) -> ("error out"=w102:errorcluster, "register values"=w39:u16[], "Modbus master out"=w86:refnum<class "Modbus Master.lvclass">)  [unwired: 5 in]
  n6 = call "Wago Input Output Converter.vi"("Input to Output?"=TRUE, "Input Command"="Ring 3") -> ("Read Input Command Location"=w62:i32)  [unwired: 9 in]
  n7 = call "UTILITY Modbus 1bit Number Combine.vi"("register values"=w39) -> ("Data"=w30:u16)  [unwired: 10 in]
  n8 = call-dynamic "Read Holding Registers.vi"("error in"=w102, "number of inputs"=u16 1, "starting address"=w62, "Modbus master in"=w86) -> ("error out"=w101:errorcluster, "register values"=w38:u16[], "Modbus master out"=w85:refnum<class "Modbus Master.lvclass">)  [unwired: 5 in]
  n9 = call "Wago Input Output Converter.vi"("Input to Output?"=TRUE, "Input Command"="Ring 4") -> ("Read Input Command Location"=w59:i32)  [unwired: 9 in]
  n10 = call "UTILITY Modbus 1bit Number Combine.vi"("register values"=w38) -> ("Data"=w29:u16)  [unwired: 10 in]
  n11 = call-dynamic "Read Holding Registers.vi"("error in"=w101, "number of inputs"=u16 1, "starting address"=w59, "Modbus master in"=w85) -> ("error out"=w100:errorcluster, "register values"=w37:u16[], "Modbus master out"=w84:refnum<class "Modbus Master.lvclass">)  [unwired: 5 in]
  n12 = call "Wago Input Output Converter.vi"("Input to Output?"=TRUE, "Input Command"="Ring 5") -> ("Read Input Command Location"=w56:i32)  [unwired: 9 in]
  n13 = call "UTILITY Modbus 1bit Number Combine.vi"("register values"=w37) -> ("Data"=w28:u16)  [unwired: 10 in]
  n14 = call-dynamic "Read Holding Registers.vi"("error in"=w100, "number of inputs"=u16 1, "starting address"=w56, "Modbus master in"=w84) -> ("error out"=w99:errorcluster, "register values"=w36:u16[], "Modbus master out"=w83:refnum<class "Modbus Master.lvclass">)  [unwired: 5 in]
  n15 = call "Wago Input Output Converter.vi"("Input to Output?"=TRUE, "Input Command"="Ring 6") -> ("Read Input Command Location"=w53:i32)  [unwired: 9 in]
  n16 = call "UTILITY Modbus 1bit Number Combine.vi"("register values"=w36) -> ("Data"=w27:u16)  [unwired: 10 in]
  n17 = call-dynamic "Read Holding Registers.vi"("error in"=w99, "number of inputs"=u16 1, "starting address"=w53, "Modbus master in"=w83) -> ("error out"=w98:errorcluster, "register values"=w35:u16[], "Modbus master out"=w82:refnum<class "Modbus Master.lvclass">)  [unwired: 5 in]
  n18 = call "Wago Input Output Converter.vi"("Input to Output?"=TRUE, "Input Command"="Ring 7") -> ("Read Input Command Location"=w50:i32)  [unwired: 9 in]
  n19 = call "UTILITY Modbus 1bit Number Combine.vi"("register values"=w35) -> ("Data"=w26:u16)  [unwired: 10 in]
  n20 = call-dynamic "Read Holding Registers.vi"("error in"=w98, "number of inputs"=u16 1, "starting address"=w50, "Modbus master in"=w82) -> ("error out"=w97:errorcluster, "register values"=w34:u16[], "Modbus master out"=w81:refnum<class "Modbus Master.lvclass">)  [unwired: 5 in]
  n21 = call "Wago Input Output Converter.vi"("Input to Output?"=TRUE, "Input Command"="Ring 8") -> ("Read Input Command Location"=w47:i32)  [unwired: 9 in]
  n22 = call "UTILITY Modbus 1bit Number Combine.vi"("register values"=w34) -> ("Data"=w25:u16)  [unwired: 10 in]
  n23 = call-dynamic "Read Holding Registers.vi"("error in"=w97, "number of inputs"=u16 1, "starting address"=w47, "Modbus master in"=w81) -> ("error out"=w96:errorcluster, "register values"=w33:u16[], "Modbus master out"=w80:refnum<class "Modbus Master.lvclass">)  [unwired: 5 in]
  n24 = call "Wago Input Output Converter.vi"("Input to Output?"=TRUE, "Input Command"="Ring 9") -> ("Read Input Command Location"=w44:i32)  [unwired: 9 in]
  n25 = call "UTILITY Modbus 1bit Number Combine.vi"("register values"=w33) -> ("Data"=w24:u16)  [unwired: 10 in]
  n26 = call-dynamic "Read Holding Registers.vi"("error in"=w96, "number of inputs"=u16 1, "starting address"=w44, "Modbus master in"=w80) -> ("error out"=w95:errorcluster, "register values"=w32:u16[], "Modbus master out"=w79:refnum<class "Modbus Master.lvclass">)  [unwired: 5 in]
  n27 = call "UTILITY Modbus 1bit Number Combine.vi"("register values"=w32) -> ("Data"=w23:u16)  [unwired: 10 in]
  n28 = call "Wago Input Output Converter.vi"("Input to Output?"=TRUE, "Input Command"="Ring 10") -> ("Read Input Command Location"=w41:i32)  [unwired: 9 in]
  n29 = call-dynamic "Read Holding Registers.vi"("error in"=w95, "number of inputs"=u16 1, "starting address"=w41, "Modbus master in"=w79) -> ("error out"=→"Error Out":errorcluster, "register values"=w22:u16[], "Modbus master out"=→"Modbus Master out":refnum<class "Modbus Master.lvclass">)  [unwired: 5 in]
  n30 = call "UTILITY Modbus 1bit Number Combine.vi"("register values"=w22) -> ("Data"=w21:u16)  [unwired: 10 in]
  n31 = Bundle By Name(cluster="Wago Data Input", "Input Process Image.Software Constants.Room PID Settings.Room Dry P(*RM Dry P1)"=w31, "Input Process Image.Software Constants.Room PID Settings.Room Dry I (*RM Dry I1)"=w30, "Input Process Image.Software Constants.Room PID Settings.Room Humidity P (*RM Hum P1)"=w29, "Input Process Image.Software Constants.Room PID Settings.Room Humidity I (*RM Hum I1)"=w28, "Input Process Image.Software Constants.Room PID Settings.Room Heat P (*RM Heat P1)"=w27, "Input Process Image.Software Constants.Room PID Settings.Room Heat I (*RM Heat I1)"=w26, "Input Process Image.Software Constants.Room PID Settings.Room Cool Temperature P (*RM Cool P1)"=w25, "Input Process Image.Software Constants.Room PID Settings.Room Cool Temperature I (*RM Cool I1)"=w24, "Input Process Image.Software Constants.Room PID Settings.Room Dehumid Temperature P (*RM Dehum P1)"=w23, "Input Process Image.Software Constants.Room PID Settings.Room Dehumid Temperature I (*RM Dehum I1)"=w21) -> (w11:T2)
  n32 = Unbundle By Name(w11) -> ("System Send Data"=w18:string[][], "Input Process Image.Software Constants.Room PID Settings.Room Dry P(*RM Dry P1)"=w13:u16, "Input Process Image.Software Constants.Room PID Settings.Room Dry I (*RM Dry I1)"=w10:u16, "Input Process Image.Software Constants.Room PID Settings.Room Humidity P (*RM Hum P1)"=w9:u16, "Input Process Image.Software Constants.Room PID Settings.Room Humidity I (*RM Hum I1)"=w8:u16, "Input Process Image.Software Constants.Room PID Settings.Room Heat P (*RM Heat P1)"=w7:u16, "Input Process Image.Software Constants.Room PID Settings.Room Heat I (*RM Heat I1)"=w6:u16, "Input Process Image.Software Constants.Room PID Settings.Room Cool Temperature P (*RM Cool P1)"=w5:u16, "Input Process Image.Software Constants.Room PID Settings.Room Cool Temperature I (*RM Cool I1)"=w4:u16, "Input Process Image.Software Constants.Room PID Settings.Room Dehumid Temperature P (*RM Dehum P1)"=w3:u16, "Input Process Image.Software Constants.Room PID Settings.Room Dehumid Temperature I (*RM Dehum I1)"=w2:u16)  [unwired: 1 out]
  n33 = Build Array(w13, w10, w9, w8, w7, w6, w5, w4, w3, w2) -> (w14:u16[])
  n34 = call "UTILITY 1D DBL to 1D String.vi"("DBL?"=FALSE, "1D DBL"=w14) -> ("1D String"=w16:string[])  [unwired: 9 in]
  n35 = Build Array(string[] ["Room Dry P", "Room Dry I", "Room Humidity P", "Room Humidity I", "Room Heat P", "Room Heat I", "Room Cool Temperature P", "Room Cool Temperature I", "Room Dehumidification Temperature P", "Room Dehumidification Temperature I"], w16) -> (w17:string[][])
  n36 = Transpose 2D Array(2D array=w17) -> (transposed array=w19:string[][])
  n37 = Build Array (concatenate)(w18, w19) -> (w20:string[][])
  n38 = Bundle By Name(cluster=w11, "System Send Data"=w20) -> (→"Wago Data Output":T2)
